vi "Record Swerve Angles.vi"(10 "Flip Motors?":bool[](array[boolean]), 11 "Angles":dbl[](array[numeric])) -> ()   [LabVIEW 2016]
uses:
  Swerve Global Variables.vi
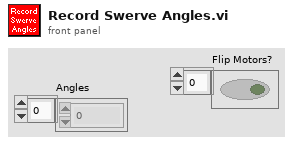
[diagram p1: front panel]
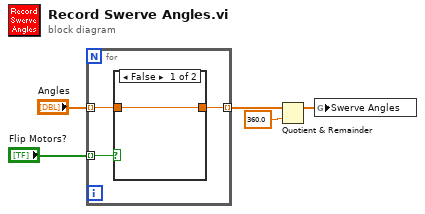
[diagram p0: block diagram]
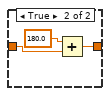
[diagram p2: hidden frame]
diagram:
  n1 = for {
    tunnel: "Angles" -> [w7] mode=indexing
    tunnel: "Flip Motors?" -> [w8] mode=indexing
    tunnel: [w6] -> w3 mode=indexing
    n2 = case shown="False" w8 {
      tunnel: w7 -> [w9 w12]
      tunnel: [w9 w10] -> w6
      frame False {
      }
      frame True {
        n3 = Add(x=180.0, y=w12) -> (x+y=w10:dbl)
      }
    }
  }
  n4 = Quotient & Remainder(x=w3, y=360.0) -> (x-y*floor(x/y)=w1:dbl[])  [unwired: 1 out]
  n5 = global write "Swerve Global Variables.vi" "Swerve Angles"(w1) -> ()
